vi "SetMeasureFilterCount.vi"(7 "SMU":T1, 8 "Error In":errorcluster, 10 "Count":u32, 11 "Keithley 2602 In":refnum<visa-resource-name>) -> (0 "Error Out":errorcluster, 3 "Keithley 2602 Out":refnum<visa-resource-name>)   [LabVIEW 2012, in "Keithley-2602.lvlib"]
uses:
  Keithley-2602.lvlib
  Controls/SMU.ctl
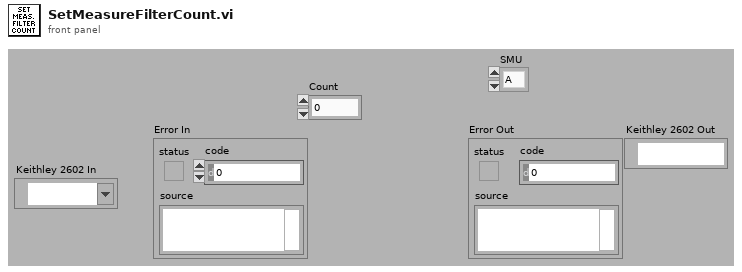
[diagram p1: front panel]
types:
  T1 = typedef "Keithley-2602.lvlib/SMU.ctl" = enum16{"A", "B"}
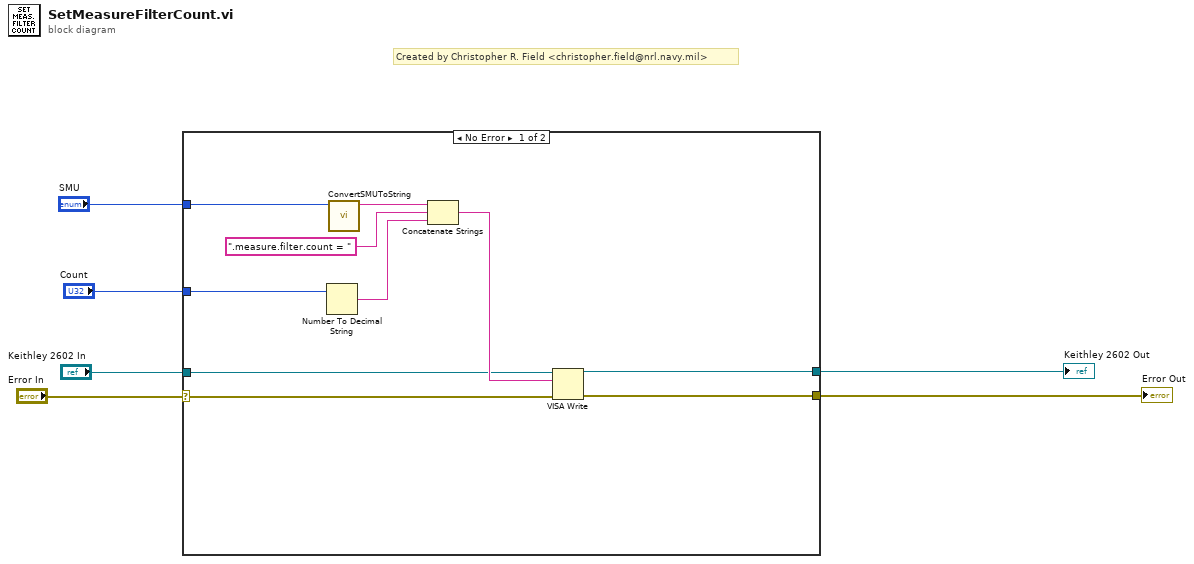
[diagram p0: block diagram]
diagram:
  # "Created by Christopher R. Field <christopher.field@nrl.navy.mil>"
  n1 = case shown="No Error" "Error In" {
    selector: "Error In" -> [w7 w17]
    tunnel: "Keithley 2602 In" -> [w13 w18]
    tunnel: [w12 w17] -> w5
    tunnel: [w11 w18] -> w4
    tunnel: "Count" -> [w10 _]
    tunnel: "SMU" -> [w8 _]
    frame No Error {
      n2 = Number To Decimal String(number=w10) -> (decimal integer string=w9:string)  [unwired: 1 in]
      n3 = call "ConvertSMUToString.vi"("SMU"=w8) -> ("Channel"=w16:string)  [unwired: 10 in]
      n4 = Concatenate Strings(w16, ".measure.filter.count = ", w9) -> (w14:string)
      n5 = VISA Write(VISA resource name=w13, write buffer=w14, error in (no error)=w7) -> (VISA resource name out=w11:refnum<visa-resource-name>, error out=w12:errorcluster)  [unwired: 1 out]
    }
    frame Error {
    }
  }
  "Error Out" <- w5
  "Keithley 2602 Out" <- w4
